vi "benchmark-list.vi"() -> ()   [LabVIEW 2017]
uses:
  c133460f-0aec-4b14-aa01-684956f011bf.vi
  679e9543-87f0-4a91-8f0b-568c5a8b50fd.vi
  TagContainer/_Support/_NameCacher.vi
  TagContainer/_Support/_datatypeChecker.vi
  TagContainer/_Support/_Ref To DVR.vi
  <vilib>/Utility/Data Type/Get Type Information.vi
  <vilib>/Utility/error.llb/Trim Whitespace.vi
  TagContainer/TagContainer.lvlib
panel:
  out "length":i32=1170
  out "unit":cluster{dbl[]}[](graph)=[{[0.0, 0.0, 0.0, 0.0, 0.0, 0.0, 0.0, 0.001003265380859375, 0.0, 0.0, 0.0, 0.0, 0.0, 0.0, 0.0, 0.0, 0.0, 0.0, 0.0, 0.0, 0.0, 0.0, 0.0, 0.0, 0.0, 0.0, 0.0, 0.0, 0.0, 0.0, 0.0, 0.0, 0.0, 0.0, 0.0, 0.0, 0.0, 0.0, 0.0, 0.0, 0.0, 0.0, 0.0, 0.0, 0.0010042190551757812, 0.0, 0.0, 0.0, 0.0, 0.0, 0.0, 0.0, 0.0, 0.0, 0.0, 0.0, 0.0, 0.0, 0.0, 0.0, 0.0, 0.0, 0.0, 0.0, 0.0, 0.0, 0.0, 0.0, 0.0, 0.0, 0.0, 0.0, 0.0, 0.0, 0.0, 0.0, 0.0, 0.0, 0.0, 0.0, 0.0010008811950683594, 0.0, 0.0, 0.0, 0.0, 0.0, 0.0, 0.0, 0.0, 0.0, 0.0, 0.0, 0.0, 0.0, 0.0, 0.0, 0.0, 0.0, 0.0, 0.0]}, {[0.0030078887939453125, 0.0, 0.0, 0.0010023117065429688, 0.0, 0.0010023117065429688, 0.0, 0.0, 0.001003265380859375, 0.0, 0.0010023117065429688, 0.0, 0.0, 0.0010023117065429688, 0.0, 0.001003265380859375, 0.0, 0.0, 0.0010023117065429688, 0.0, 0.0010027885437011719, 0.0, 0.0, 0.0010027885437011719, 0.0, 0.0010018348693847656, 0.0, 0.0, 0.001003265380859375, 0.0, 0.0010023117065429688, 0.0, 0.0, 0.0010023117065429688, 0.0, 0.001003265380859375, 0.0, 0.0, 0.001003265380859375, 0.0, 0.0010013580322265625, 0.0, 0.0, 0.001003265380859375, 0.0, 0.0010023117065429688, 0.0, 0.0, 0.0010027885437011719, 0.0, 0.0010023117065429688, 0.0, 0.0, 0.001003265380859375, 0.0, 0.0010023117065429688, 0.0, 0.0, 0.0010023117065429688, 0.0, 0.0010023117065429688, 0.0, 0.0, 0.001003265380859375, 0.0, 0.0010023117065429688, 0.0, 0.0, 0.0010027885437011719, 0.0, 0.0010027885437011719, 0.0, 0.0, 0.0010027885437011719, 0.0, 0.0010023117065429688, 0.0, 0.0, 0.0010023117065429688, 0.0, 0.001003265380859375, 0.0, 0.0, 0.0010023117065429688, 0.0, 0.0010023117065429688, 0.0, 0.0, 0.0010023117065429688, 0.0, 0.001003265380859375, 0.0, 0.0, 0.0010023117065429688, 0.0, 0.0010027885437011719, 0.0, 0.0, 0.0010027885437011719, 0.0]}]
  out "outside":i32=99
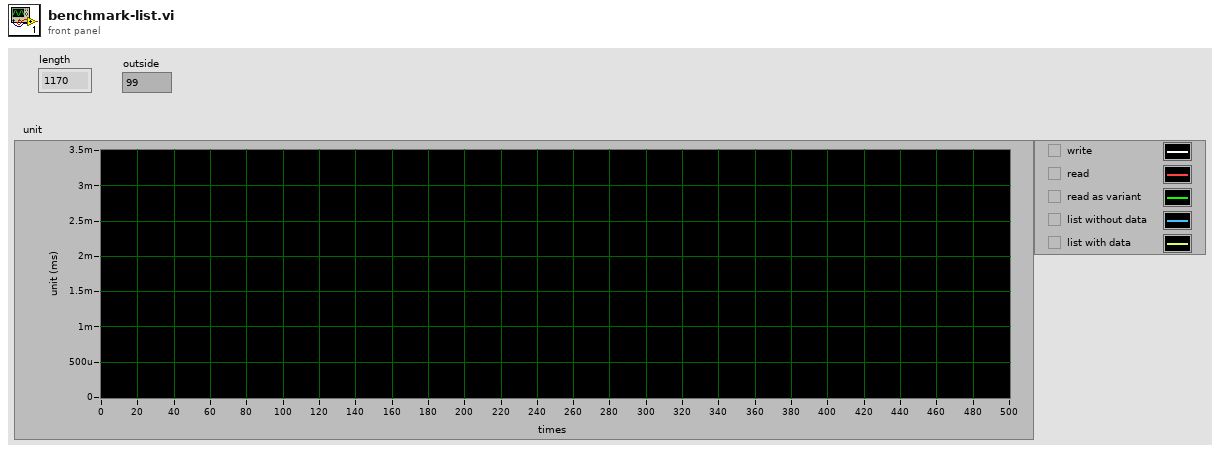
[diagram p1: front panel]
types:
  T1 = cluster{"error constant":errorcluster, "error constant 2":errorcluster, "error constant 3":errorcluster, "error constant 4":errorcluster, "error constant 5":errorcluster, "error constant 6":errorcluster, "error constant 7":errorcluster, "error constant 8":errorcluster, "error constant 9":errorcluster, "error constant 10":errorcluster, "error constant 11":errorcluster, "error constant 12":errorcluster, "error constant 13":errorcluster, "error constant 14":errorcluster, "error constant 15":errorcluster, "error constant 16":errorcluster, "error constant 17":errorcluster, "error constant 18":errorcluster, "error constant 19":errorcluster, "error constant 20":errorcluster, "error constant 21":errorcluster, "error constant 22":errorcluster, "error constant 23":errorcluster, "error constant 24":errorcluster, "error constant 25":errorcluster, "error constant 26":errorcluster, "error constant 27":errorcluster, "error constant 28":errorcluster, "error constant 29":errorcluster, "error constant 30":errorcluster, "error constant 31":errorcluster, "error constant 32":errorcluster, "error constant 33":errorcluster, "error constant 34":errorcluster, "error constant 35":errorcluster, "error constant 36":errorcluster, "error constant 37":errorcluster, "error constant 38":errorcluster, "error constant 39":errorcluster, "error constant 40":errorcluster, "error constant 41":errorcluster, "error constant 42":errorcluster, "error constant 43":errorcluster, "error constant 44":errorcluster, "error constant 45":errorcluster, "error constant 46":errorcluster, "error constant 47":errorcluster, "error constant 48":errorcluster, "error constant 49":errorcluster, "error constant 50":errorcluster, "error constant 51":errorcluster, "error constant 52":errorcluster, "error constant 53":errorcluster, "error constant 54":errorcluster, "error constant 55":errorcluster, "error constant 56":errorcluster, "error constant 57":errorcluster, "error constant 58":errorcluster, "error constant 59":errorcluster, "error constant 60":errorcluster, "error constant 61":errorcluster, "error constant 62":errorcluster, "error constant 63":errorcluster, "error constant 64":errorcluster, "error constant 65":errorcluster, cluster{"error constant":errorcluster, "error constant 2":errorcluster, "error constant 3":errorcluster, "error constant 4":errorcluster, "error constant 5":errorcluster, "error constant 6":errorcluster, "error constant 7":errorcluster, "error constant 8":errorcluster, "error constant 9":errorcluster, "error constant 10":errorcluster, "error constant 11":errorcluster, "error constant 12":errorcluster, "error constant 13":errorcluster, "error constant 14":errorcluster, "error constant 15":errorcluster, "error constant 16":errorcluster, "error constant 17":errorcluster, "error constant 18":errorcluster, "error constant 19":errorcluster, "error constant 20":errorcluster, "error constant 21":errorcluster, "error constant 22":errorcluster, "error constant 23":errorcluster, "error constant 24":errorcluster, "error constant 25":errorcluster, "error constant 26":errorcluster, "error constant 27":errorcluster, "error constant 28":errorcluster, "error constant 29":errorcluster, "error constant 30":errorcluster, "error constant 31":errorcluster, "error constant 32":errorcluster, "error constant 33":errorcluster, "error constant 34":errorcluster, "error constant 35":errorcluster, "error constant 36":errorcluster, "error constant 37":errorcluster, "error constant 38":errorcluster, "error constant 39":errorcluster, "error constant 40":errorcluster, "error constant 41":errorcluster, "error constant 42":errorcluster, "error constant 43":errorcluster, "error constant 44":errorcluster, "error constant 45":errorcluster, "error constant 46":errorcluster, "error constant 47":errorcluster, "error constant 48":errorcluster, "error constant 49":errorcluster, "error constant 50":errorcluster, "error constant 51":errorcluster, "error constant 52":errorcluster, "error constant 53":errorcluster, "error constant 54":errorcluster, "error constant 55":errorcluster, "error constant 56":errorcluster, "error constant 57":errorcluster, "error constant 58":errorcluster, "error constant 59":errorcluster, "error constant 60":errorcluster, "error constant 61":errorcluster, "error constant 62":errorcluster, "error constant 63":errorcluster, "error constant 64":errorcluster, "error constant 65":errorcluster}}
  T2 = typedef "TagContainer.lvlib/TagContainer.ctl" = refnum<k1>
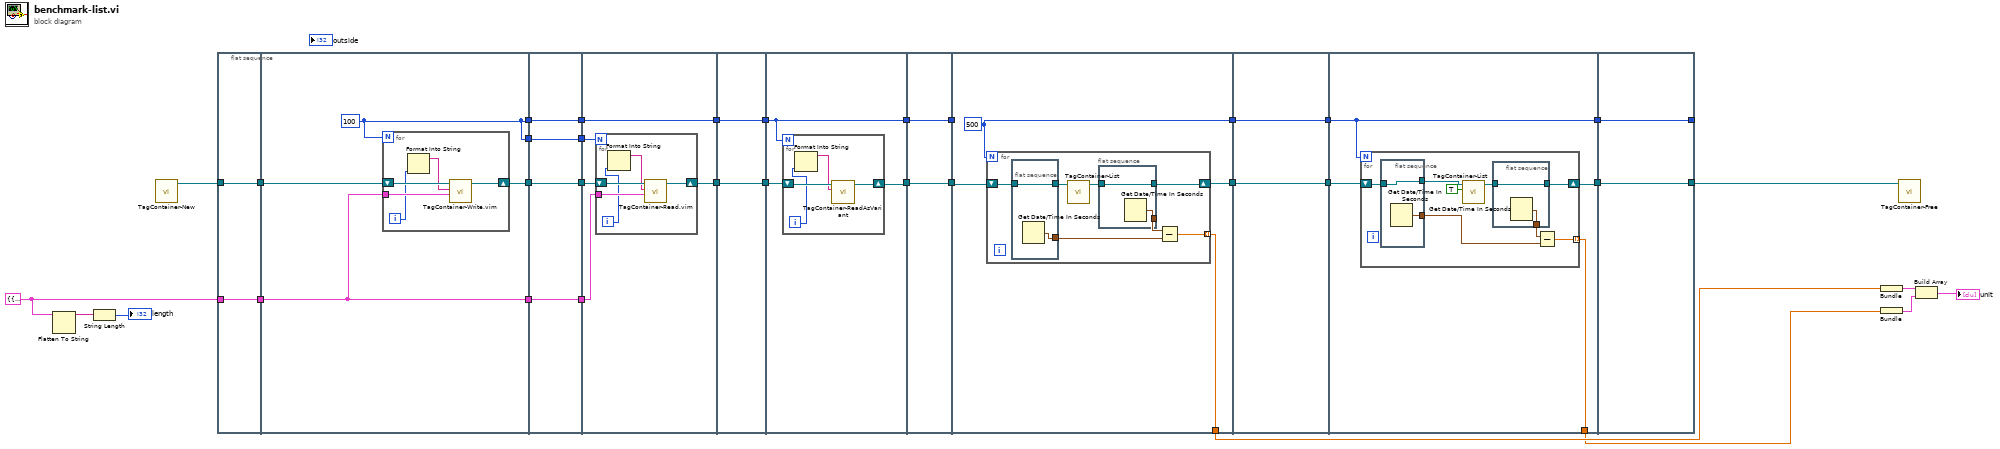
[diagram p0: block diagram]
diagram:
  w31 = T1 {"error constant"={"status"=FALSE, "code"=0, "source"=""}, "error constant 2"={"status"=FALSE, "code"=0, "source"=""}, "error constant 3"={"status"=FALSE, "code"=0, "source"=""}, "error constant 4"={"status"=FALSE, "code"=0, "source"=""}, "error constant 5"={"status"=FALSE, "code"=0, "source"=""}, "error constant 6"={"status"=FALSE, "code"=0, "source"=""}, "error constant 7"={"status"=FALSE, "code"=0, "source"=""}, "error constant 8"={"status"=FALSE, "code"=0, "source"=""}, "error constant 9"={"status"=FALSE, "code"=0, "source"=""}, "error constant 10"={"status"=FALSE, "code"=0, "source"=""}, "error constant 11"={"status"=FALSE, "code"=0, "source"=""}, "error constant 12"={"status"=FALSE, "code"=0, "source"=""}, "error constant 13"={"status"=FALSE, "code"=0, "source"=""}, "error constant 14"={"status"=FALSE, "code"=0, "source"=""}, "error constant 15"={"status"=FALSE, "code"=0, "source"=""}, "error constant 16"={"status"=FALSE, "code"=0, "source"=""}, "error constant 17"={"status"=FALSE, "code"=0, "source"=""}, "error constant 18"={"status"=FALSE, "code"=0, "source"=""}, "error constant 19"={"status"=FALSE, "code"=0, "source"=""}, "error constant 20"={"status"=FALSE, "code"=0, "source"=""}, "error constant 21"={"status"=FALSE, "code"=0, "source"=""}, "error constant 22"={"status"=FALSE, "code"=0, "source"=""}, "error constant 23"={"status"=FALSE, "code"=0, "source"=""}, "error constant 24"={"status"=FALSE, "code"=0, "source"=""}, "error constant 25"={"status"=FALSE, "code"=0, "source"=""}, "error constant 26"={"status"=FALSE, "code"=0, "source"=""}, "error constant 27"={"status"=FALSE, "code"=0, "source"=""}, "error constant 28"={"status"=FALSE, "code"=0, "source"=""}, "error constant 29"={"status"=FALSE, "code"=0, "source"=""}, "error constant 30"={"status"=FALSE, "code"=0, "source"=""}, "error constant 31"={"status"=FALSE, "code"=0, "source"=""}, "error constant 32"={"status"=FALSE, "code"=0, "source"=""}, "error constant 33"={"status"=FALSE, "code"=0, "source"=""}, "error constant 34"={"status"=FALSE, "code"=0, "source"=""}, "error constant 35"={"status"=FALSE, "code"=0, "source"=""}, "error constant 36"={"status"=FALSE, "code"=0, "source"=""}, "error constant 37"={"status"=FALSE, "code"=0, "source"=""}, "error constant 38"={"status"=FALSE, "code"=0, "source"=""}, "error constant 39"={"status"=FALSE, "code"=0, "source"=""}, "error constant 40"={"status"=FALSE, "code"=0, "source"=""}, "error constant 41"={"status"=FALSE, "code"=0, "source"=""}, "error constant 42"={"status"=FALSE, "code"=0, "source"=""}, "error constant 43"={"status"=FALSE, "code"=0, "source"=""}, "error constant 44"={"status"=FALSE, "code"=0, "source"=""}, "error constant 45"={"status"=FALSE, "code"=0, "source"=""}, "error constant 46"={"status"=FALSE, "code"=0, "source"=""}, "error constant 47"={"status"=FALSE, "code"=0, "source"=""}, "error constant 48"={"status"=FALSE, "code"=0, "source"=""}, "error constant 49"={"status"=FALSE, "code"=0, "source"=""}, "error constant 50"={"status"=FALSE, "code"=0, "source"=""}, "error constant 51"={"status"=FALSE, "code"=0, "source"=""}, "error constant 52"={"status"=FALSE, "code"=0, "source"=""}, "error constant 53"={"status"=FALSE, "code"=0, "source"=""}, "error constant 54"={"status"=FALSE, "code"=0, "source"=""}, "error constant 55"={"status"=FALSE, "code"=0, "source"=""}, "error constant 56"={"status"=FALSE, "code"=0, "source"=""}, "error constant 57"={"status"=FALSE, "code"=0, "source"=""}, "error constant 58"={"status"=FALSE, "code"=0, "source"=""}, "error constant 59"={"status"=FALSE, "code"=0, "source"=""}, "error constant 60"={"status"=FALSE, "code"=0, "source"=""}, "error constant 61"={"status"=FALSE, "code"=0, "source"=""}, "error constant 62"={"status"=FALSE, "code"=0, "source"=""}, "error constant 63"={"status"=FALSE, "code"=0, "source"=""}, "error constant 64"={"status"=FALSE, "code"=0, "source"=""}, "error constant 65"={"status"=FALSE, "code"=0, "source"=""}, {"error constant"={"status"=FALSE, "code"=0, "source"=""}, "error constant 2"={"status"=FALSE, "code"=0, "source"=""}, "error constant 3"={"status"=FALSE, "code"=0, "source"=""}, "error constant 4"={"status"=FALSE, "code"=0, "source"=""}, "error constant 5"={"status"=FALSE, "code"=0, "source"=""}, "error constant 6"={"status"=FALSE, "code"=0, "source"=""}, "error constant 7"={"status"=FALSE, "code"=0, "source"=""}, "error constant 8"={"status"=FALSE, "code"=0, "source"=""}, "error constant 9"={"status"=FALSE, "code"=0, "source"=""}, "error constant 10"={"status"=FALSE, "code"=0, "source"=""}, "error constant 11"={"status"=FALSE, "code"=0, "source"=""}, "error constant 12"={"status"=FALSE, "code"=0, "source"=""}, "error constant 13"={"status"=FALSE, "code"=0, "source"=""}, "error constant 14"={"status"=FALSE, "code"=0, "source"=""}, "error constant 15"={"status"=FALSE, "code"=0, "source"=""}, "error constant 16"={"status"=FALSE, "code"=0, "source"=""}, "error constant 17"={"status"=FALSE, "code"=0, "source"=""}, "error constant 18"={"status"=FALSE, "code"=0, "source"=""}, "error constant 19"={"status"=FALSE, "code"=0, "source"=""}, "error constant 20"={"status"=FALSE, "code"=0, "source"=""}, "error constant 21"={"status"=FALSE, "code"=0, "source"=""}, "error constant 22"={"status"=FALSE, "code"=0, "source"=""}, "error constant 23"={"status"=FALSE, "code"=0, "source"=""}, "error constant 24"={"status"=FALSE, "code"=0, "source"=""}, "error constant 25"={"status"=FALSE, "code"=0, "source"=""}, "error constant 26"={"status"=FALSE, "code"=0, "source"=""}, "error constant 27"={"status"=FALSE, "code"=0, "source"=""}, "error constant 28"={"status"=FALSE, "code"=0, "source"=""}, "error constant 29"={"status"=FALSE, "code"=0, "source"=""}, "error constant 30"={"status"=FALSE, "code"=0, "source"=""}, "error constant 31"={"status"=FALSE, "code"=0, "source"=""}, "error constant 32"={"status"=FALSE, "code"=0, "source"=""}, "error constant 33"={"status"=FALSE, "code"=0, "source"=""}, "error constant 34"={"status"=FALSE, "code"=0, "source"=""}, "error constant 35"={"status"=FALSE, "code"=0, "source"=""}, "error constant 36"={"status"=FALSE, "code"=0, "source"=""}, "error constant 37"={"status"=FALSE, "code"=0, "source"=""}, "error constant 38"={"status"=FALSE, "code"=0, "source"=""}, "error constant 39"={"status"=FALSE, "code"=0, "source"=""}, "error constant 40"={"status"=FALSE, "code"=0, "source"=""}, "error constant 41"={"status"=FALSE, "code"=0, "source"=""}, "error constant 42"={"status"=FALSE, "code"=0, "source"=""}, "error constant 43"={"status"=FALSE, "code"=0, "source"=""}, "error constant 44"={"status"=FALSE, "code"=0, "source"=""}, "error constant 45"={"status"=FALSE, "code"=0, "source"=""}, "error constant 46"={"status"=FALSE, "code"=0, "source"=""}, "error constant 47"={"status"=FALSE, "code"=0, "source"=""}, "error constant 48"={"status"=FALSE, "code"=0, "source"=""}, "error constant 49"={"status"=FALSE, "code"=0, "source"=""}, "error constant 50"={"status"=FALSE, "code"=0, "source"=""}, "error constant 51"={"status"=FALSE, "code"=0, "source"=""}, "error constant 52"={"status"=FALSE, "code"=0, "source"=""}, "error constant 53"={"status"=FALSE, "code"=0, "source"=""}, "error constant 54"={"status"=FALSE, "code"=0, "source"=""}, "error constant 55"={"status"=FALSE, "code"=0, "source"=""}, "error constant 56"={"status"=FALSE, "code"=0, "source"=""}, "error constant 57"={"status"=FALSE, "code"=0, "source"=""}, "error constant 58"={"status"=FALSE, "code"=0, "source"=""}, "error constant 59"={"status"=FALSE, "code"=0, "source"=""}, "error constant 60"={"status"=FALSE, "code"=0, "source"=""}, "error constant 61"={"status"=FALSE, "code"=0, "source"=""}, "error constant 62"={"status"=FALSE, "code"=0, "source"=""}, "error constant 63"={"status"=FALSE, "code"=0, "source"=""}, "error constant 64"={"status"=FALSE, "code"=0, "source"=""}, "error constant 65"={"status"=FALSE, "code"=0, "source"=""}}}
  n1 = Flatten To String(anything=w31) -> (data string=w30:string)  [unwired: 3 in, 2 out]
  n2 = String Length(string=w30) -> (length=→"length":i32)
  n3 = call "TagContainer-New.vi"() -> ("TagContainer"=w33:T2)  [unwired: 10 in, 1 out]
  n4 = flat-sequence {
    tunnel: [w36] -> w29
    tunnel: [w35] -> w28
    tunnel: w33 -> [w36]
    tunnel: w31 -> [w35]
    tunnel: [w38] -> w27
    tunnel: [w39] -> w26
    tunnel: w29 -> [w40]
    tunnel: w28 -> [w37]
    tunnel: [w38] -> w25
    tunnel: [w37] -> w24
    tunnel: w27 -> [w49]
    tunnel: [w49] -> w23
    tunnel: [w48] -> w22
    tunnel: w26 -> [w48]
    tunnel: w25 -> [w47]
    tunnel: [w47] -> w21
    tunnel: [w46] -> w20
    tunnel: w24 -> [w46]
    tunnel: w23 -> [w54]
    tunnel: w22 -> [w53]
    tunnel: [w54] -> w19
    tunnel: [w52] -> w18
    tunnel: w21 -> [w51]
    tunnel: w20 -> [w50]
    tunnel: w19 -> [w61]
    tunnel: w18 -> [w60]
    tunnel: [w61] -> w17
    tunnel: [w60] -> w16
    tunnel: w17 -> [w63]
    tunnel: [w63] -> w15
    tunnel: [w64] -> w14
    tunnel: w16 -> [w62]
    tunnel: w15 -> [w70]
    tunnel: w14 -> [w69]
    tunnel: [w70] -> w13
    tunnel: [w69] -> w12
    tunnel: w13 -> [_]
    tunnel: w12 -> [w74]
    tunnel: [w71] -> w11
    tunnel: [w73] -> w10
    tunnel: [w72] -> w5
    tunnel: w11 -> [w87]
    tunnel: w10 -> [w86]
    tunnel: [w87] -> w9
    tunnel: [w86] -> w8
    tunnel: w9 -> [w89]
    tunnel: w8 -> [w91]
    tunnel: [w89] -> w7
    tunnel: [w90] -> w6
    tunnel: [w88] -> w4
    tunnel: [w104] -> w32
    tunnel: [w105] -> _
    tunnel: w7 -> [w105]
    tunnel: w6 -> [w104]
    frame #0 {
    }
    frame #1 {
      w38 = 100
      n5 = for {
        N: w38 -> [_]
        tunnel: w37 -> [w43]
        shift-right: [w44] -> w39
        shift-left: w40 -> [w45]
        i -> [w41]
        n6 = Format Into String(w41) -> (resulting string=w42:string)  [unwired: 3 in, 1 out]
        n7 = call "TagContainer-Write.vim"("Value"=w43, "name"=w42, "TagContainer"=w45) -> ("TagContainer(dup)"=w44:T2)  [unwired: 7 in, 1 out]
      }
    }
    frame #2 {
    }
    frame #3 {
      n8 = for {
        N: w51 -> [_]
        shift-right: [w58] -> w52
        shift-left: w53 -> [w59]
        tunnel: w50 -> [w56]
        i -> [w55]
        n9 = Format Into String(w55) -> (resulting string=w57:string)  [unwired: 3 in, 1 out]
        n10 = call "TagContainer-Read.vim"("Type"=w56, "name"=w57, "TagContainer"=w59) -> ("TagContainer(dup)"=w58:T2)  [unwired: 3 in, 5 out]
      }
    }
    frame #4 {
    }
    frame #5 {
      n11 = for {
        N: w63 -> [_]
        shift-right: [w67] -> w64
        shift-left: w62 -> [w68]
        i -> [w65]
        n12 = Format Into String(w65) -> (resulting string=w66:string)  [unwired: 3 in, 1 out]
        n13 = call "TagContainer-ReadAsVariant.vi"("name"=w66, "TagContainer"=w68) -> ("TagContainer(dup)"=w67:T2)  [unwired: 4 in, 5 out]
      }
    }
    frame #6 {
    }
    frame #7 {
      w71 = 500
      n14 = for {
        N: w71 -> [_]
        shift-right: [w76] -> w73
        shift-left: w74 -> [w77]
        tunnel: [w79] -> w72 mode=indexing
        n15 = flat-sequence {
          tunnel: [w85] -> w80
          tunnel: [w84] -> w78
          tunnel: w77 -> [w84]
          frame #0 {
            n16 = Get Date/Time In Seconds() -> (seconds since 1Jan1904=w85:timestamp)
          }
        }
        n17 = call "TagContainer-List.vi"("TagContainer"=w78) -> ("TagContainer(dup)"=w75:T2)  [unwired: 7 in, 3 out]
        n18 = flat-sequence {
          tunnel: [w83] -> w81
          tunnel: [w82] -> w76
          tunnel: w75 -> [w82]
          frame #0 {
            n19 = Get Date/Time In Seconds() -> (seconds since 1Jan1904=w83:timestamp)
          }
        }
        n20 = Subtract(x=w81, y=w80) -> (x-y=w79:dbl)
      }
    }
    frame #8 {
    }
    frame #9 {
      n21 = for {
        N: w89 -> [_]
        shift-right: [w93] -> w90
        shift-left: w91 -> [w94]
        tunnel: [w96] -> w88 mode=indexing
        n22 = flat-sequence {
          tunnel: [w103] -> w97
          tunnel: [w102] -> w95
          tunnel: w94 -> [w102]
          frame #0 {
            n23 = Get Date/Time In Seconds() -> (seconds since 1Jan1904=w103:timestamp)
          }
        }
        n24 = call "TagContainer-List.vi"("with Data?(F)"=TRUE, "TagContainer"=w95) -> ("TagContainer(dup)"=w92:T2)  [unwired: 6 in, 3 out]
        n25 = flat-sequence {
          tunnel: [w101] -> w98
          tunnel: [w100] -> w93
          tunnel: w92 -> [w100]
          frame #0 {
            n26 = Get Date/Time In Seconds() -> (seconds since 1Jan1904=w101:timestamp)
          }
        }
        n27 = Subtract(x=w98, y=w97) -> (x-y=w96:dbl)
      }
    }
    frame #10 {
    }
  }
  n28 = Bundle(w5) -> (w3:cluster{dbl[]})  [unwired: 1 in]
  n29 = Bundle(w4) -> (w2:cluster{dbl[]})  [unwired: 1 in]
  n30 = call "TagContainer-Free.vi"("TagContainer"=w32) -> ()  [unwired: 10 in, 1 out]
  n31 = Build Array(w3, w2) -> (→"unit":cluster{dbl[]}[])
